vi "Encode Channels.vi"(6 "Offset":i32, 8 "error in":errorcluster, 9 "Parameters":T2(array[cluster]) {"encoding" items=["BNR", "BCD", "Discrete", "Signed_32", "Signed_64", "Float_32", "Float_64", "Opaque"]}, 10 "Data in":u8[](array[numeric]), 11 "Values in":dbl[](array[numeric])) -> (0 "error out":errorcluster, 2 "Data out":u8[](array[numeric]), 4 "Number of Parameters":i32)   [LabVIEW 2020]
uses:
  b24d3698-aaae-4200-bf93-4b6af5480478.vi
  5b1080be-549e-4688-aad8-fb955257d8ef.vi
  7e7e8f0d-6015-4215-b4f4-37ecf7ce16f3.vi
  7b487445-4b60-493e-9c15-0f5b7677c2b1.vi
  f46899e6-f3c2-4da0-acc2-ed34a334556c.vi
  2afa5e5b-ae47-4ac6-b34f-e51087edfaba.vi
  1eaed3cb-9180-4944-bca4-c812fd7aad88.vi
  Encoding (Arinc664).ctl
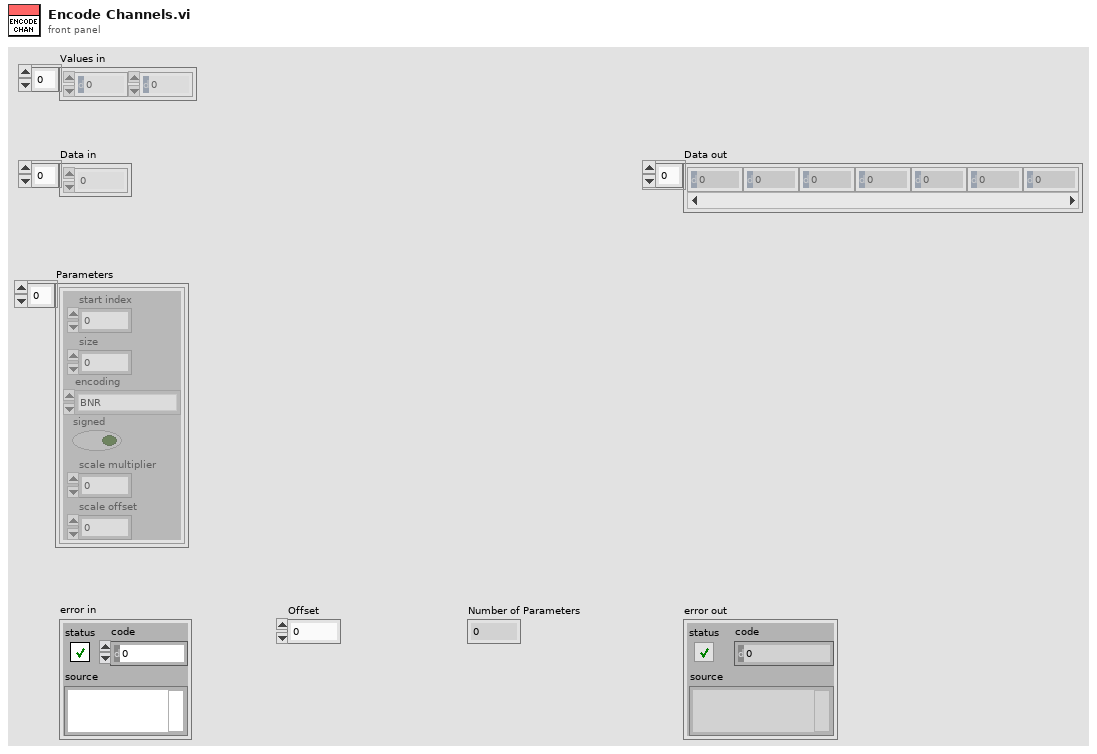
[diagram p1: front panel]
types:
  T1 = typedef "Encoding (Arinc664).ctl" = u16
  T2 = cluster{"start index":i32, "size":i32, "encoding":T1, "signed":bool, "scale multiplier":dbl, "scale offset":dbl}[]
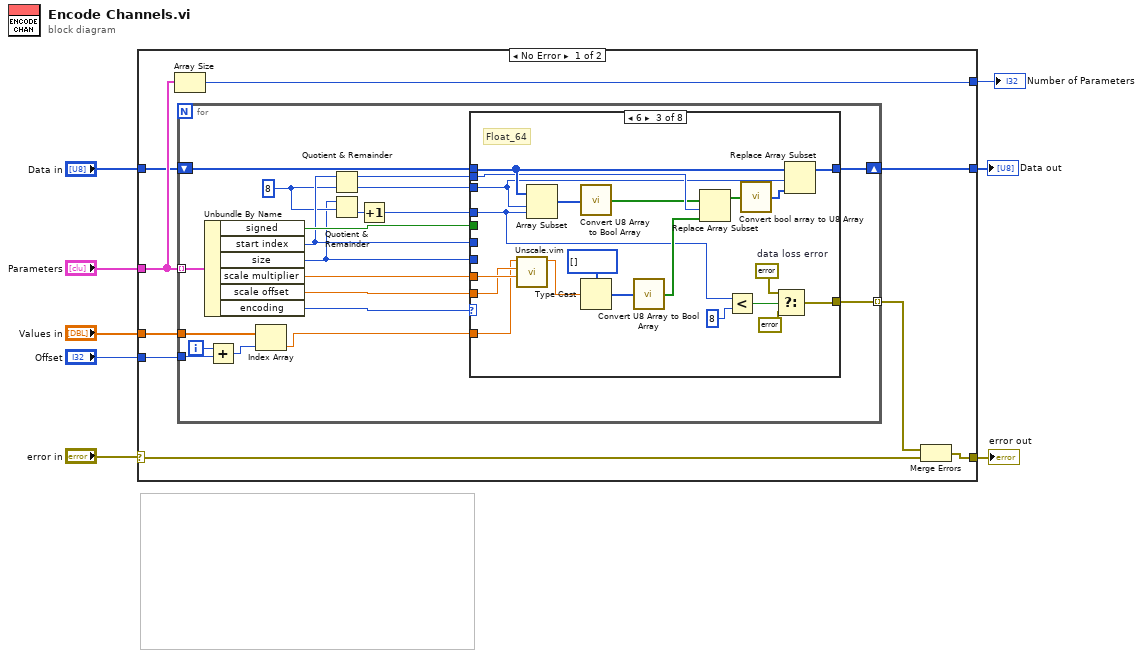
[diagram p0: block diagram]
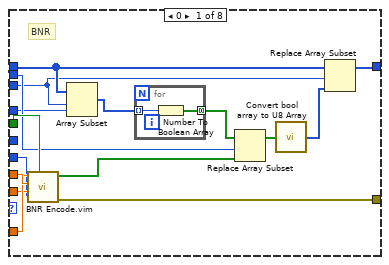
[diagram p2: hidden frame]
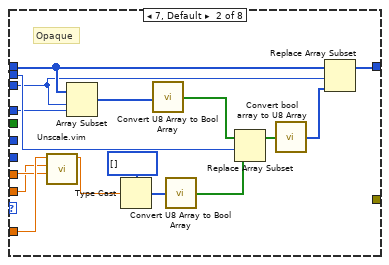
[diagram p3: hidden frame]
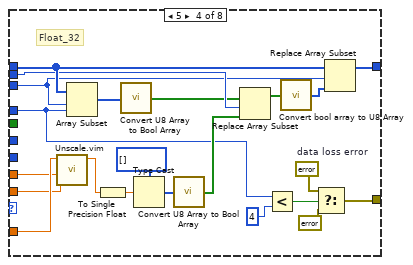
[diagram p4: hidden frame]
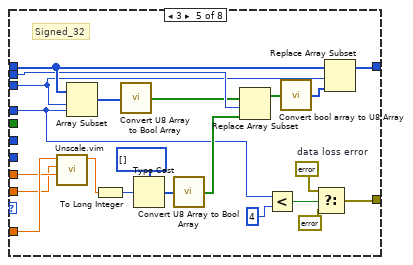
[diagram p5: hidden frame]
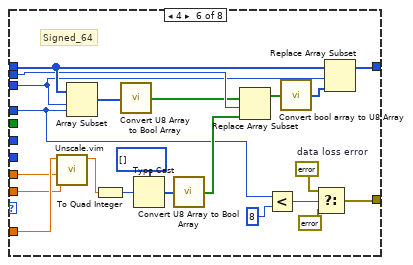
[diagram p6: hidden frame]
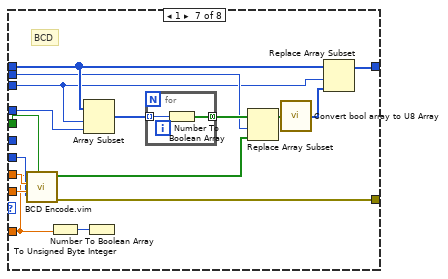
[diagram p7: hidden frame]
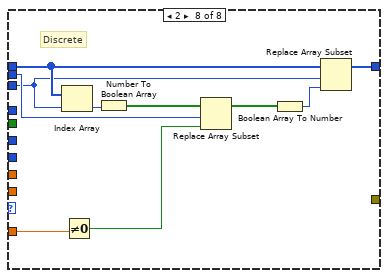
[diagram p8: hidden frame]
diagram:
  n1 = case shown="No Error" "error in" {
    selector: "error in" -> [w13 w189]
    tunnel: "Values in" -> [w17 _]
    tunnel: [w16 w188] -> w7
    tunnel: [w14 w189] -> w5
    tunnel: "Offset" -> [w12 _]
    tunnel: [w11 _] -> w3
    tunnel: "Parameters" -> [w10 _]
    tunnel: "Data in" -> [w9 w188]
    frame No Error {
      n2 = Array Size(array=w10) -> (size(s)=w11:i32)
      n3 = for {
        tunnel: w17 -> [w35]
        tunnel: w10 -> [w36] mode=indexing
        shift-right: [w34] -> w16
        shift-left: w9 -> [w37]
        tunnel: [w33] -> w15 mode=indexing
        tunnel: w12 -> [w31]
        i -> [w32]
        w23 = 8 ("y")
        n4 = Unbundle By Name(w36) -> ("signed"=w25:bool, "start index"=w24:i32, "size"=w22:i32, "scale multiplier"=w27:dbl, "scale offset"=w26:dbl, "encoding"=w28:T1)
        n5 = Add(x=w32, y=w31) -> (x+y=w30:i32)
        n6 = Index Array(array=w35, index=w30) -> (element=w29:dbl)
        n7 = Quotient & Remainder(x=w24, y=w23) -> (x-y*floor(x/y)=w20:i32, floor(x/y)=w21:i32)
        n8 = Quotient & Remainder(x=w22, y=w23) -> (floor(x/y)=w19:i32)  [unwired: 1 out]
        n9 = Increment(x=w19) -> (x+1=w18:i32)
        n10 = case shown="6" w28 {
          tunnel: w25 -> [w53 _ _ _ _ _ w175 _]
          tunnel: w27 -> [w52 w63 w86 w107 w129 w151 w174 _]
          tunnel: w26 -> [w50 w62 w85 w106 w128 w150 w173 _]
          tunnel: w37 -> [w48 w71 w92 w114 w136 w158 w171 w187]
          tunnel: w24 -> [_ _ _ _ _ _ _ _]
          tunnel: w22 -> [w49 _ _ _ _ _ w172 _]
          tunnel: w29 -> [w51 w64 w73 w108 w130 w152 w163 w182]
          tunnel: [w46 w69 w90 w112 w134 w156 w170 w186] -> w34
          tunnel: w21 -> [w38 w65 w87 w109 w131 w153 w159 w179]
          tunnel: w20 -> [w47 w70 w91 w113 w135 w157 w160 w183]
          tunnel: w18 -> [w43 w68 w76 w96 w118 w140 w167 _]
          tunnel: [w39 _ w78 w98 w120 w142 w164 _] -> w33
          frame 0 {
            # "BNR"
            n11 = call "BNR Encode.vim"("data size (bits)"=w49, "signed"=w53, "scale offset"=w50, "scale multiplier"=w52, "value"=w51) -> ("error out"=w39:errorcluster, "BNR encoded value"=w42:bool[])  [unwired: 5 in]
            n12 = Array Subset(array=w48, index=w38, length=w43) -> (w45:u8[])
            n13 = for {
              tunnel: w45 -> [w55] mode=indexing
              tunnel: [w54] -> w44 mode=concatenating
              n14 = Number To Boolean Array(number=w55) -> (Boolean array=w54:bool[])
            }
            n15 = Replace Array Subset(array=w44, new element=w42, index=w47) -> (w41:bool[])
            n16 = call "Convert bool array to U8 Array.vi"("Boolean array"=w41) -> ("Array"=w40:u8[])  [unwired: 14 in]
            n17 = Replace Array Subset(array=w48, new element=w40, index=w38) -> (w46:u8[])
          }
          frame 7, Default {
            # "Opaque"
            n18 = call "Unscale.vim"("scale multiplier"=w63, "scale offset"=w62, "value"=w64) -> ("unscaled value"=w61:dbl)  [unwired: 8 in]
            n19 = Array Subset(array=w71, index=w65, length=w68) -> (w59:u8[])
            n20 = Type Cast(type=u8[] [] ("subarray"), x=w61) -> (*(type *) &x=w57:u8[])
            n21 = call "Convert U8 Array to Bool Array.vi"("U8 array in"=w59) -> ("Boolean array out"=w58:bool[])  [unwired: 14 in]
            n22 = call "Convert U8 Array to Bool Array.vi"("U8 array in"=w57) -> ("Boolean array out"=w56:bool[])  [unwired: 14 in]
            n23 = Replace Array Subset(array=w58, new element=w56, index=w70) -> (w67:bool[])
            n24 = call "Convert bool array to U8 Array.vi"("Boolean array"=w67) -> ("Array"=w66:u8[])  [unwired: 14 in]
            n25 = Replace Array Subset(array=w71, new element=w66, index=w65) -> (w69:u8[])
          }
          frame 6 {
            w79 = errorcluster {"status"=TRUE, "code"=-732301, "source"="data loss during encoding"}  # data loss error
            # "Float_64"
            n26 = call "Unscale.vim"("scale multiplier"=w86, "scale offset"=w85, "value"=w73) -> ("unscaled value"=w72:dbl)  [unwired: 8 in]
            n27 = Array Subset(array=w92, index=w87, length=w76) -> (w83:u8[])
            n28 = call "Convert U8 Array to Bool Array.vi"("U8 array in"=w83) -> ("Boolean array out"=w81:bool[])  [unwired: 14 in]
            n29 = Type Cast(type=u8[] [] ("subarray"), x=w72) -> (*(type *) &x=w82:u8[])
            n30 = call "Convert U8 Array to Bool Array.vi"("U8 array in"=w82) -> ("Boolean array out"=w80:bool[])  [unwired: 14 in]
            n31 = Replace Array Subset(array=w81, new element=w80, index=w91) -> (w89:bool[])
            n32 = Less?(x=w76, y=8) -> (x < y?=w75:bool)
            n33 = call "Convert bool array to U8 Array.vi"("Boolean array"=w89) -> ("Array"=w88:u8[])  [unwired: 14 in]
            n34 = Select(t=w79, s=w75, f=errorcluster {"status"=FALSE, "code"=0, "source"=""}) -> (s? t:f=w78:errorcluster)
            n35 = Replace Array Subset(array=w92, new element=w88, index=w87) -> (w90:u8[])
          }
          frame 5 {
            w99 = errorcluster {"status"=TRUE, "code"=-732301, "source"="data loss during encoding"}  # data loss error
            # "Float_32"
            n36 = call "Unscale.vim"("scale multiplier"=w107, "scale offset"=w106, "value"=w108) -> ("unscaled value"=w105:dbl)  [unwired: 8 in]
            n37 = Array Subset(array=w114, index=w109, length=w96) -> (w103:u8[])
            n38 = To Single Precision Float(number=w105) -> (single precision float=w93:sgl)
            n39 = call "Convert U8 Array to Bool Array.vi"("U8 array in"=w103) -> ("Boolean array out"=w101:bool[])  [unwired: 14 in]
            n40 = Type Cast(type=u8[] [] ("subarray"), x=w93) -> (*(type *) &x=w102:u8[])
            n41 = call "Convert U8 Array to Bool Array.vi"("U8 array in"=w102) -> ("Boolean array out"=w100:bool[])  [unwired: 14 in]
            n42 = Replace Array Subset(array=w101, new element=w100, index=w113) -> (w111:bool[])
            n43 = Less?(x=w96, y=4) -> (x < y?=w95:bool)
            n44 = call "Convert bool array to U8 Array.vi"("Boolean array"=w111) -> ("Array"=w110:u8[])  [unwired: 14 in]
            n45 = Select(t=w99, s=w95, f=errorcluster {"status"=FALSE, "code"=0, "source"=""}) -> (s? t:f=w98:errorcluster)
            n46 = Replace Array Subset(array=w114, new element=w110, index=w109) -> (w112:u8[])
          }
          frame 3 {
            w121 = errorcluster {"status"=TRUE, "code"=-732301, "source"="data loss during encoding"}  # data loss error
            # "Signed_32"
            n47 = call "Unscale.vim"("scale multiplier"=w129, "scale offset"=w128, "value"=w130) -> ("unscaled value"=w127:dbl)  [unwired: 8 in]
            n48 = Array Subset(array=w136, index=w131, length=w118) -> (w125:u8[])
            n49 = To Long Integer(number=w127) -> (32bit integer=w115:i32)
            n50 = call "Convert U8 Array to Bool Array.vi"("U8 array in"=w125) -> ("Boolean array out"=w123:bool[])  [unwired: 14 in]
            n51 = Type Cast(type=u8[] [] ("subarray"), x=w115) -> (*(type *) &x=w124:u8[])
            n52 = call "Convert U8 Array to Bool Array.vi"("U8 array in"=w124) -> ("Boolean array out"=w122:bool[])  [unwired: 14 in]
            n53 = Replace Array Subset(array=w123, new element=w122, index=w135) -> (w133:bool[])
            n54 = Less?(x=w118, y=4) -> (x < y?=w117:bool)
            n55 = call "Convert bool array to U8 Array.vi"("Boolean array"=w133) -> ("Array"=w132:u8[])  [unwired: 14 in]
            n56 = Select(t=w121, s=w117, f=errorcluster {"status"=FALSE, "code"=0, "source"=""}) -> (s? t:f=w120:errorcluster)
            n57 = Replace Array Subset(array=w136, new element=w132, index=w131) -> (w134:u8[])
          }
          frame 4 {
            w143 = errorcluster {"status"=TRUE, "code"=-732301, "source"="data loss during encoding"}  # data loss error
            # "Signed_64"
            n58 = call "Unscale.vim"("scale multiplier"=w151, "scale offset"=w150, "value"=w152) -> ("unscaled value"=w149:dbl)  [unwired: 8 in]
            n59 = Array Subset(array=w158, index=w153, length=w140) -> (w147:u8[])
            n60 = To Quad Integer(1:w149) -> (0:w137:i64)
            n61 = call "Convert U8 Array to Bool Array.vi"("U8 array in"=w147) -> ("Boolean array out"=w145:bool[])  [unwired: 14 in]
            n62 = Type Cast(type=u8[] [] ("subarray"), x=w137) -> (*(type *) &x=w146:u8[])
            n63 = call "Convert U8 Array to Bool Array.vi"("U8 array in"=w146) -> ("Boolean array out"=w144:bool[])  [unwired: 14 in]
            n64 = Replace Array Subset(array=w145, new element=w144, index=w157) -> (w155:bool[])
            n65 = Less?(x=w140, y=8) -> (x < y?=w139:bool)
            n66 = call "Convert bool array to U8 Array.vi"("Boolean array"=w155) -> ("Array"=w154:u8[])  [unwired: 14 in]
            n67 = Select(t=w143, s=w139, f=errorcluster {"status"=FALSE, "code"=0, "source"=""}) -> (s? t:f=w142:errorcluster)
            n68 = Replace Array Subset(array=w158, new element=w154, index=w153) -> (w156:u8[])
          }
          frame 1 {
            # "BCD"
            n69 = call "BCD Encode.vim"("data size (bits)"=w172, "signed"=w175, "scale offset"=w173, "scale multiplier"=w174, "value"=w163) -> ("error out"=w164:errorcluster, "BCD encoded value"=w161:bool[])  [unwired: 4 in, 1 out]
            n70 = To Unsigned Byte Integer(number=w163) -> (unsigned 8bit integer=w162:u8)
            n71 = Array Subset(array=w171, index=w159, length=w167) -> (w169:u8[])
            n72 = Number To Boolean Array(number=w162) -> ()  [unwired: 1 out]
            n73 = for {
              tunnel: w169 -> [w177] mode=indexing
              tunnel: [w176] -> w168 mode=concatenating
              n74 = Number To Boolean Array(number=w177) -> (Boolean array=w176:bool[])
            }
            n75 = Replace Array Subset(array=w168, new element=w161, index=w160) -> (w166:bool[])
            n76 = call "Convert bool array to U8 Array.vi"("Boolean array"=w166) -> ("Array"=w165:u8[])  [unwired: 14 in]
            n77 = Replace Array Subset(array=w171, new element=w165, index=w159) -> (w170:u8[])
          }
          frame 2 {
            # "Discrete"
            n78 = Index Array(array=w187, index=w179) -> (element=w185:u8)
            n79 = Not Equal To 0?(x=w182) -> (x != 0?=w181:bool)
            n80 = Number To Boolean Array(number=w185) -> (Boolean array=w184:bool[])
            n81 = Replace Array Subset(array=w184, new element=w181, index=w183) -> (w180:bool[])
            n82 = Boolean Array To Number(Boolean array=w180) -> (number=w178:u32)
            n83 = Replace Array Subset(array=w187, new element=w178, index=w179) -> (w186:u8[])
          }
        }
      }
      n84 = Merge Errors(w15, w13) -> (w14:errorcluster)
    }
    frame Error {
    }
  }
  "Data out" <- w7
  "error out" <- w5
  "Number of Parameters" <- w3
